vi "Send Message.vi"(6 "timeout (100)":i32=100, 8 "error in (no error)":errorcluster, 9 "Message Data":string, 10 "Message":string, 11 "Master CR in":refnum<class "Master CR.lvclass">) -> (0 "error out":errorcluster, 1 "timed out?":bool, 3 "Master CR out":refnum<class "Master CR.lvclass">)   [LabVIEW 2021, in "Master CR.lvclass"]
uses:
  Master CR.lvclass
  Master CR.lvclass/Master CR.ctl
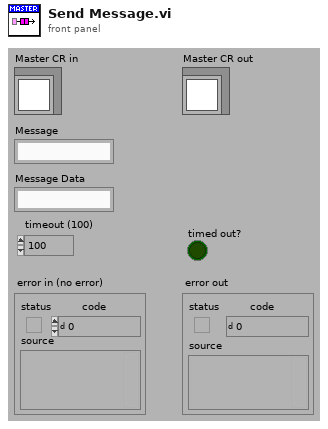
[diagram p1: front panel]
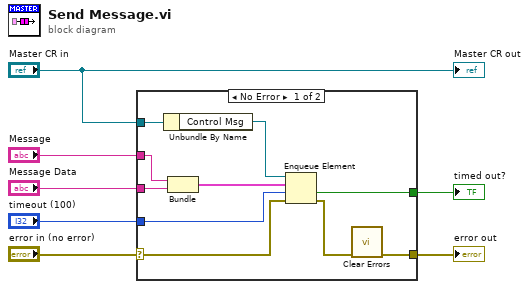
[diagram p0: block diagram]
diagram:
  n1 = case shown="No Error" "error in (no error)" {
    selector: "error in (no error)" -> [w17 w18]
    tunnel: [w8 w18] -> w7
    tunnel: "timeout (100)" -> [w11 _]
    tunnel: [w15 _] -> w4
    tunnel: "Master CR in" -> [w9 _]
    tunnel: "Message" -> [w13 _]
    tunnel: "Message Data" -> [w14 _]
    frame No Error {
      n2 = Unbundle By Name(w9) -> ("Control Msg"=w16:refnum<queue>)
      n3 = Bundle("Message"=w13, "Message Data"=w14) -> (w12:cluster{"Message":string, "Message Data":string})  [unwired: 1 in]
      n4 = Enqueue Element(queue=w16, element=w12, timeout in ms (-1)=w11, error in (no error)=w17) -> (timed out?=w15:bool, error out=w10:errorcluster)  [unwired: 1 out]
      n5 = call <vilib>:"Clear Errors.vi"("error in (no error)"=w10) -> ("error out"=w8:errorcluster)  [unwired: 5 in, 1 out]
    }
    frame Error {
    }
  }
  "error out" <- w7
  "timed out?" <- w4
  "Master CR out" <- "Master CR in"
